vi "CreateBuffer.vi"(8 "error in (no error)":errorcluster, 9 "Buffer size":i32, 10 "Data type":T2(ring)=enum."I16") -> (0 "error out":errorcluster, 2 "Pointer and BufferSize":u64[](array[numeric]))   [LabVIEW 2024]
uses:
  <vilib>/Utility/error.llb/DialogType.ctl
panel:
  in  "type of dialog (OK msg:1)":T1=4 items=["no dialog", "OK message", "continue or stop message", "OK message + warnings", "continue/stop + warnings"]
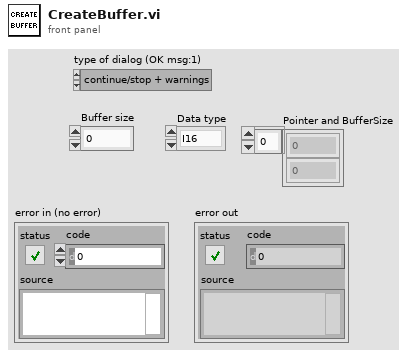
[diagram p1: front panel]
types:
  T1 = typedef "DialogType.ctl" = u16
  T2 = enum16{"U8", "I8", "U16", "I16", "U32", "I32", "U64", "I64"}
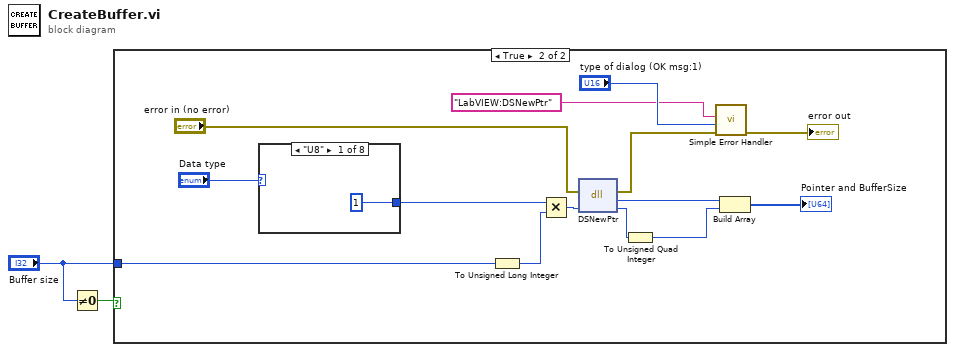
[diagram p0: block diagram]
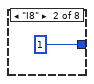
[diagram p3: hidden frame]
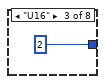
[diagram p4: hidden frame]
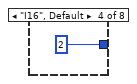
[diagram p5: hidden frame]
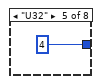
[diagram p6: hidden frame]
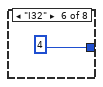
[diagram p7: hidden frame]
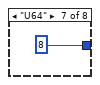
[diagram p8: hidden frame]
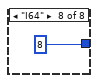
[diagram p9: hidden frame]
diagram:
  n1 = Not Equal To 0?(x="Buffer size") -> (x != 0?=w1:bool)
  n2 = case shown="True" w1 {
    tunnel: "Buffer size" -> [_ w10]
    frame False {
    }
    frame True {
      n3 = case shown="\"U8\"" "Data type" {
        tunnel: [u32 1 ("element") u32 1 ("element") u32 2 ("element") u32 2 ("element") u32 4 ("element") u32 4 ("element") u32 8 ("element") u32 8 ("element")] -> w7
        frame "U8" {
        }
        frame "I8" {
        }
        frame "U16" {
        }
        frame "I16", Default {
        }
        frame "U32" {
        }
        frame "I32" {
        }
        frame "U64" {
        }
        frame "I64" {
        }
      }
      n4 = To Unsigned Long Integer(number=w10) -> (unsigned 32bit integer=w12:u32)
      n5 = Multiply(x=w7, y=w12) -> (x*y=w16:u32)
      n6 = dll-call lib="LabVIEW" fn="DSNewPtr"(error in="error in (no error)", "Size"=w16) -> (error out=w6:errorcluster, "Pointer"=w15:u64, "Size"=w14:u32)  [unwired: 2 in, 1 out]
      n7 = To Unsigned Quad Integer(1:w14) -> (0:w13:u64)
      n8 = call <vilib>:"Simple Error Handler.vi"("error source (\" \")"="LabVIEW:DSNewPtr", "type of dialog (OK msg:1)"="type of dialog (OK msg:1)", "error in (no error)"=w6) -> ("error out"=→"error out":errorcluster)  [unwired: 2 in, 4 out]
      n9 = Build Array(w15, w13) -> (→"Pointer and BufferSize":u64[])
    }
  }
